vi "FRCts20_EspEngine_SetSearchBrowser.vi"(8 "error in (no error)":errorcluster, 10 "SearchBrowser":T1, 11 "httpRequestID":u32) -> (0 "error out":errorcluster, 2 "SearchBrowser":T1, 3 "httpRequestID out":u32)   [LabVIEW 2014, in "FRCts20_EspEngine.lvlib"]
uses:
  FRCts20_EspEngine.lvlib
  TypeDefs/FRCts20_EspEngine_SearchBrowser.ctl
  <vilib>/wsapi/subVIs/Set String ESP Variable.vi
  <vilib>/wsapi/NI_WebServices.lvlib
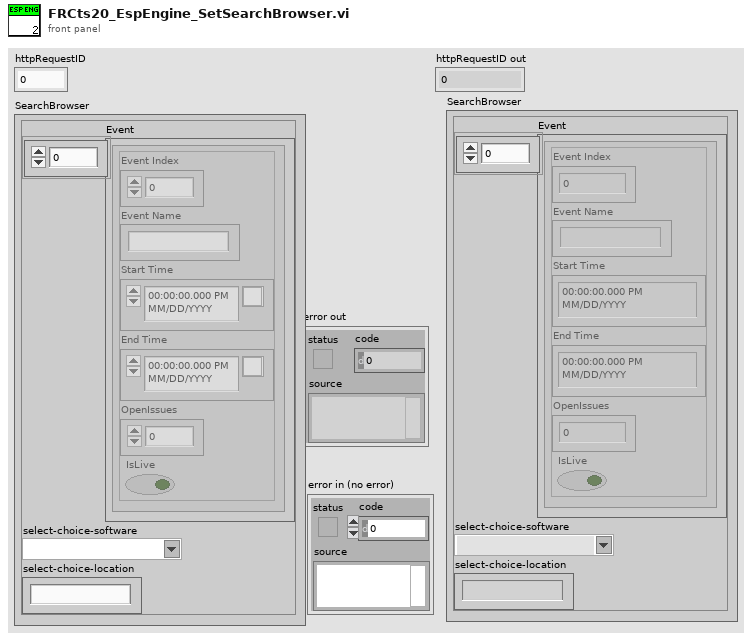
[diagram p1: front panel]
types:
  T1 = typedef "FRCts20_EspEngine.lvlib/FRCts20_EspEngine_SearchBrowser.ctl" = cluster{"Event":cluster{"Event Index":u32, "Event Name":string, "Start Time":timestamp, "End Time":timestamp, "OpenIssues":u8, "IsLive":bool}[], "select-choice-software":string, "select-choice-location":string}
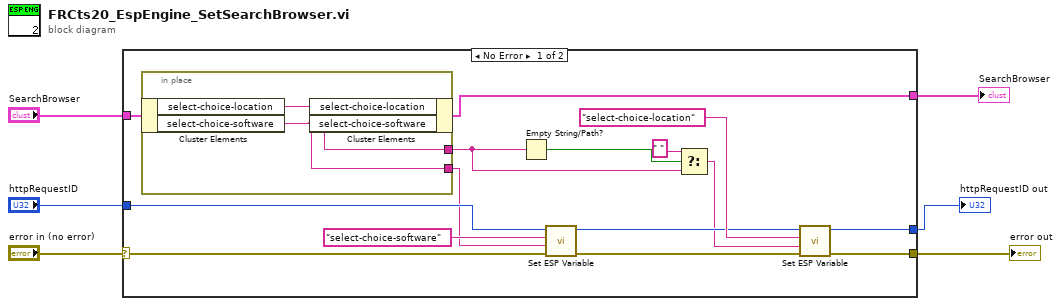
[diagram p0: block diagram]
diagram:
  n1 = case shown="No Error" "error in (no error)" {
    selector: "error in (no error)" -> [w11 w24]
    tunnel: [w13 w24] -> w6
    tunnel: "httpRequestID" -> [w12 _]
    tunnel: [w21 _] -> w3
    tunnel: "SearchBrowser" -> [w10 _]
    tunnel: [w7 _] -> w1
    frame No Error {
      n2 = in-place {
        in-place-border: [w23] -> w9
        in-place-border: [w22] -> w8
        n3 = in-place-cluster #1(w10) -> ("select-choice-location"=w23:string, "select-choice-software"=w22:string)
        n4 = in-place-cluster #1("select-choice-location"=w23, "select-choice-software"=w22) -> (w7:T1)
      }
      n5 = Empty String/Path?(string/path=w9) -> (empty?=w16:bool)
      n6 = call-poly <vilib>:"Set ESP Variable.vi"("error in (no error)"=w11, "value"=w8, "key"="select-choice-software", "httpRequestID"=w12) -> ("error out"=w17:errorcluster, "httpRequestID out"=w18:u32)  [unwired: 6 in]
      n7 = Select(t=" ", s=w16, f=w9) -> (s? t:f=w14:string)
      n8 = call-poly <vilib>:"Set ESP Variable.vi"("error in (no error)"=w17, "value"=w14, "key"="select-choice-location", "httpRequestID"=w18) -> ("error out"=w13:errorcluster, "httpRequestID out"=w21:u32)  [unwired: 6 in]
    }
    frame Error {
    }
  }
  "error out" <- w6
  "httpRequestID out" <- w3
  "SearchBrowser" <- w1
